vi "Get cif_manager_PluginInfoArray.vi"(8 "error in (no error)":errorcluster, 11 "gRPCid":T1) -> (0 "error out":errorcluster, 2 "package_templatemessage":T2, 3 "gRPCid out":T1)   [LabVIEW 2021, in "CIF_Manager_server.lvlib"]
uses:
  CIF_Manager_server.lvlib
  cif_manager_PluginInfoArray.ctl
  cif_manager_PluginInfo.ctl
  cif_common_ShortVersion.ctl
  cif_management_common_PluginStatusData.ctl
  cif_management_common_PluginStatusData_PluginState.ctl
  cif_management_common_TimingStatistics.ctl
  cif_common_TimingStats.ctl
  cif_management_common_FifoStatistics.ctl
  cif_management_common_Error.ctl
  cif_management_common_MonitorDoubles.ctl
  cif_management_common_MonitorU64.ctl
  cif_management_common_MonitorI64.ctl
  cif_management_common_LoaderInfo.ctl
  cif_management_common_LoaderType.ctl
  <vilib>/gRPC/LabVIEW gRPC Library/Shared/grpcId.ctl
  cif_manager_PluginInfoArray_Flat.ctl
  cif_manager_PluginInfo_Flat.ctl
  cif_common_ShortVersion_Flat.ctl
  cif_management_common_PluginStatusData_Flat.ctl
  cif_management_common_TimingStatistics_Flat.ctl
  cif_common_TimingStats_Flat.ctl
  cif_management_common_FifoStatistics_Flat.ctl
  cif_management_common_Error_Flat.ctl
  cif_management_common_MonitorDoubles_Flat.ctl
  cif_management_common_MonitorU64_Flat.ctl
  cif_management_common_MonitorI64_Flat.ctl
  cif_management_common_LoaderInfo_Flat.ctl
  2ed25e12-861d-4677-8ead-ace2906b2041.vi
  <vilib>/gRPC/LabVIEW gRPC Library/Shared/TranslateGrpcError.vi
  FlatToRichcif_manager_PluginInfo.vi
  FlatToRichcif_common_ShortVersion.vi
  FlatToRichcif_management_common_PluginStatusData.vi
  FlatToRichcif_management_common_LoaderInfo.vi
  FlatToRichcif_management_common_TimingStatistics.vi
  FlatToRichcif_management_common_FifoStatistics.vi
  FlatToRichcif_management_common_Error.vi
  FlatToRichcif_management_common_MonitorDoubles.vi
  FlatToRichcif_management_common_MonitorU64.vi
  FlatToRichcif_management_common_MonitorI64.vi
  FlatToRichcif_common_TimingStats.vi
  <vilib>/gRPC/LabVIEW gRPC Library/Server API/Server/Get Server DLL Path.vi
  <vilib>/Utility/error.llb/Error Cluster From Error Code.vi
  <vilib>/gRPC/LabVIEW gRPC Library/grpc-lvsupport-release.lvlib
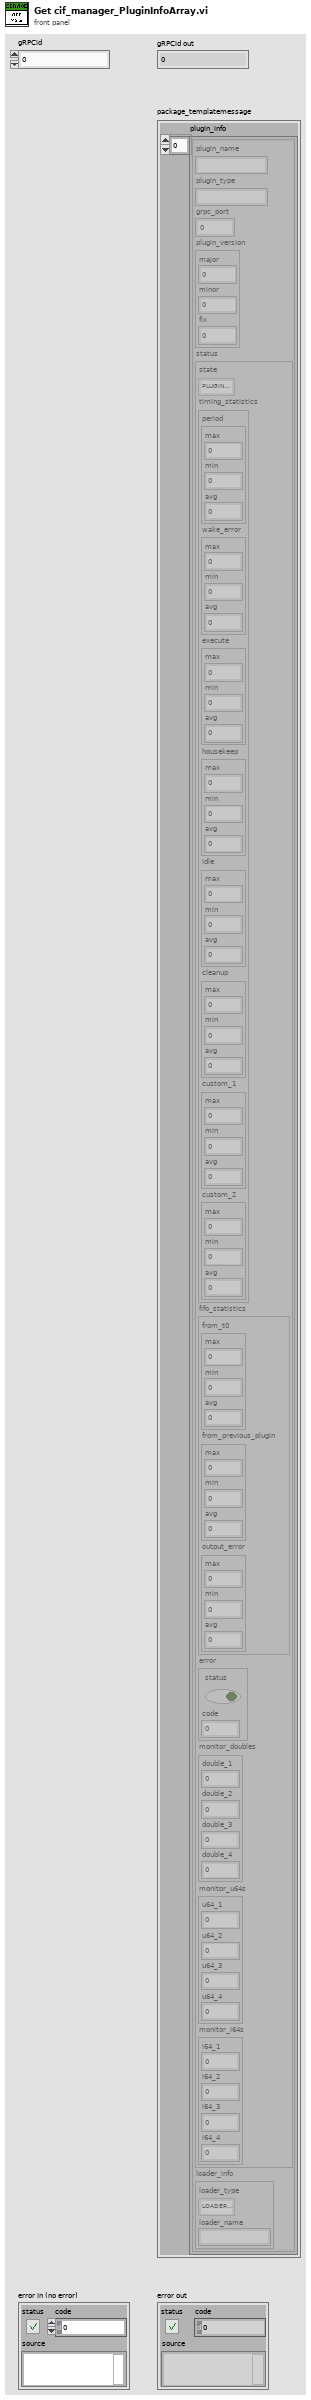
[diagram p1: front panel]
types:
  T1 = typedef "grpc-lvsupport-release.lvlib/grpcId.ctl" = u64
  T2 = typedef "CIF_Manager_server.lvlib/cif_manager_PluginInfoArray.ctl" = cluster{"plugin_info":T3[]}
  T3 = typedef "CIF_Manager_server.lvlib/cif_manager_PluginInfo.ctl" = cluster{"plugin_name":string, "plugin_type":string, "grpc_port":i32, "plugin_version":T4, "status":T5, "loader_info":T14}
  T4 = typedef "CIF_Manager_server.lvlib/cif_common_ShortVersion.ctl" = cluster{"major":u32, "minor":u32, "fix":u32}
  T5 = typedef "CIF_Manager_server.lvlib/cif_management_common_PluginStatusData.ctl" = cluster{"state":T6, "timing_statistics":T7, "fifo_statistics":T9, "error":T10, "monitor_doubles":T11, "monitor_u64s":T12, "monitor_i64s":T13}
  T6 = typedef "CIF_Manager_server.lvlib/cif_management_common_PluginStatusData_PluginState.ctl" = enum32{"PLUGINSTATE_UNKNOWN", "PLUGINSTATE_CREATING", "PLUGINSTATE_LISTENING", "PLUGINSTATE_RUNNING", "PLUGINSTATE_CLEANINGUP", "PLUGINSTATE_DESTROYING", "PLUGINSTATE_PREPARED", "PLUGINSTATE_FTE_RUN"}
  T7 = typedef "CIF_Manager_server.lvlib/cif_management_common_TimingStatistics.ctl" = cluster{"period":T8, "wake_error":T8, "execute":T8, "housekeep":T8, "idle":T8, "cleanup":T8, "custom_1":T8, "custom_2":T8}
  T8 = typedef "CIF_Manager_server.lvlib/cif_common_TimingStats.ctl" = cluster{"max":i64, "min":i64, "avg":dbl}
  T9 = typedef "CIF_Manager_server.lvlib/cif_management_common_FifoStatistics.ctl" = cluster{"from_t0":T8, "from_previous_plugin":T8, "output_error":T8}
  T10 = typedef "CIF_Manager_server.lvlib/cif_management_common_Error.ctl" = cluster{"status":bool, "code":i32}
  T11 = typedef "CIF_Manager_server.lvlib/cif_management_common_MonitorDoubles.ctl" = cluster{"double_1":dbl, "double_2":dbl, "double_3":dbl, "double_4":dbl}
  T12 = typedef "CIF_Manager_server.lvlib/cif_management_common_MonitorU64.ctl" = cluster{"u64_1":u64, "u64_2":u64, "u64_3":u64, "u64_4":u64}
  T13 = typedef "CIF_Manager_server.lvlib/cif_management_common_MonitorI64.ctl" = cluster{"i64_1":i64, "i64_2":i64, "i64_3":i64, "i64_4":i64}
  T14 = typedef "CIF_Manager_server.lvlib/cif_management_common_LoaderInfo.ctl" = cluster{"loader_type":T15, "loader_name":string}
  T15 = typedef "CIF_Manager_server.lvlib/cif_management_common_LoaderType.ctl" = enum32{"LOADERTYPE_UNKNOWN", "LOADERTYPE_LABVIEW"}
  T16 = typedef "CIF_Manager_server.lvlib/cif_manager_PluginInfoArray_Flat.ctl" = cluster{"plugin_info":T17[]}
  T17 = typedef "CIF_Manager_server.lvlib/cif_manager_PluginInfo_Flat.ctl" = cluster{"plugin_name":string, "plugin_type":string, "grpc_port":i32, "plugin_version":T18, "status":T19, "loader_info":T27}
  T18 = typedef "CIF_Manager_server.lvlib/cif_common_ShortVersion_Flat.ctl" = cluster{"major":u32, "minor":u32, "fix":u32}
  T19 = typedef "CIF_Manager_server.lvlib/cif_management_common_PluginStatusData_Flat.ctl" = cluster{"state":T6, "timing_statistics":T20, "fifo_statistics":T22, "error":T23, "monitor_doubles":T24, "monitor_u64s":T25, "monitor_i64s":T26}
  T20 = typedef "CIF_Manager_server.lvlib/cif_management_common_TimingStatistics_Flat.ctl" = cluster{"period":T21, "wake_error":T21, "execute":T21, "housekeep":T21, "idle":T21, "cleanup":T21, "custom_1":T21, "custom_2":T21}
  T21 = typedef "CIF_Manager_server.lvlib/cif_common_TimingStats_Flat.ctl" = cluster{"max":i64, "min":i64, "avg":dbl}
  T22 = typedef "CIF_Manager_server.lvlib/cif_management_common_FifoStatistics_Flat.ctl" = cluster{"from_t0":T21, "from_previous_plugin":T21, "output_error":T21}
  T23 = typedef "CIF_Manager_server.lvlib/cif_management_common_Error_Flat.ctl" = cluster{"status":bool, "code":i32}
  T24 = typedef "CIF_Manager_server.lvlib/cif_management_common_MonitorDoubles_Flat.ctl" = cluster{"double_1":dbl, "double_2":dbl, "double_3":dbl, "double_4":dbl}
  T25 = typedef "CIF_Manager_server.lvlib/cif_management_common_MonitorU64_Flat.ctl" = cluster{"u64_1":u64, "u64_2":u64, "u64_3":u64, "u64_4":u64}
  T26 = typedef "CIF_Manager_server.lvlib/cif_management_common_MonitorI64_Flat.ctl" = cluster{"i64_1":i64, "i64_2":i64, "i64_3":i64, "i64_4":i64}
  T27 = typedef "CIF_Manager_server.lvlib/cif_management_common_LoaderInfo_Flat.ctl" = cluster{"loader_type":T15, "loader_name":string}
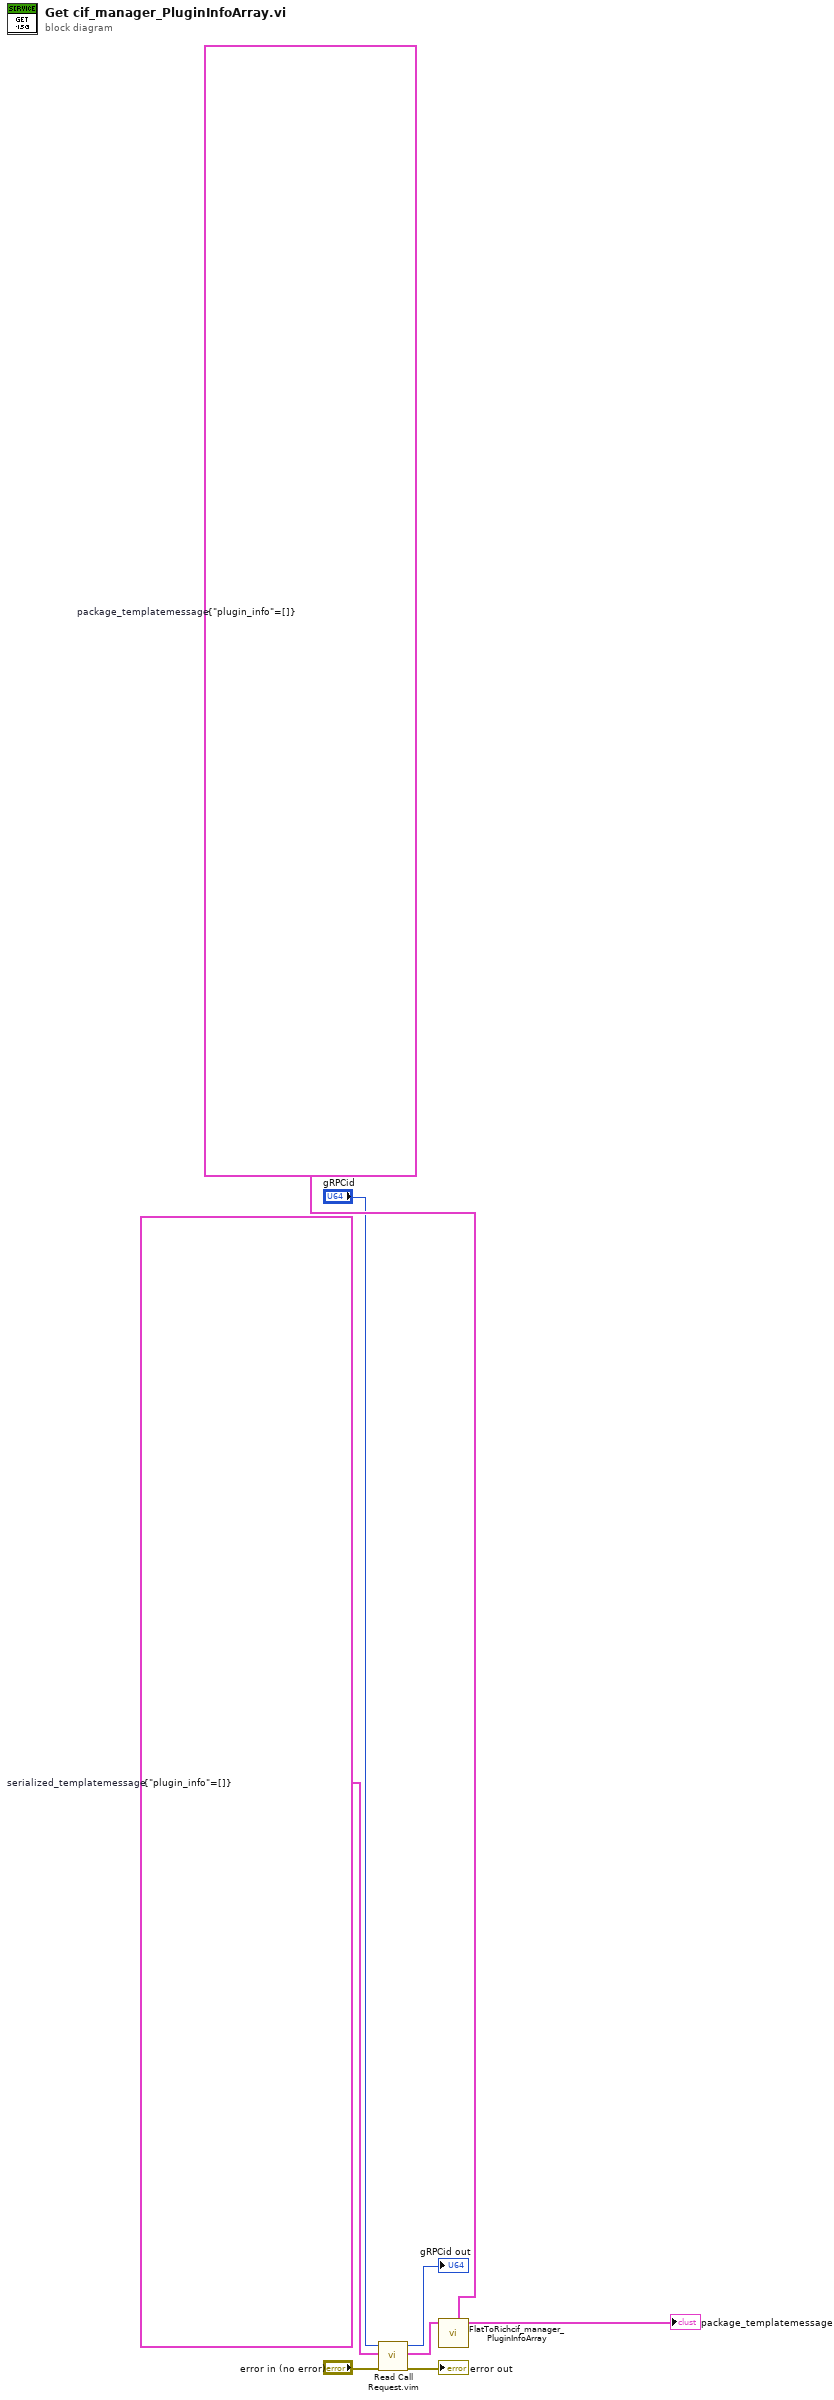
[diagram p0: block diagram]
diagram:
  w6 = T16 {"plugin_info"=[]}  # serialized_templatemessage
  w5 = T2 {"plugin_info"=[]}  # package_templatemessage
  n1 = call "Read Call Request.vim"("error in"="error in (no error)", "Request Type"=w6, "gRPCid in"="gRPCid") -> ("error out"=→"error out":errorcluster, "Request Data"=w4:T16, "gRPCid out"=→"gRPCid out":T1)  [unwired: 6 in]
  n2 = call "FlatToRichcif_manager_PluginInfoArray.vi"("OutputClusterType"=w5, "InputCluster"=w4) -> ("OutputCluster"=→"package_templatemessage":T2)  [unwired: 9 in]
